vi "Update State String.vi"(8 "error in (no error)":errorcluster, 10 "State Control":string, 11 "Chef State in":refnum<class "Chef State.lvclass">) -> (0 "error out":errorcluster, 3 "Chef State out":refnum<class "Chef State.lvclass">)   [LabVIEW 2021, in "Chef States.lvlib" / "Chef State.lvclass"]
uses:
  Chef State.lvclass
  <vilib>/ActorFramework/Actor/Actor.lvclass
  Root Actor Logic/Root Actor Logic Messages/Update State String Msg/Update State String Msg.lvclass
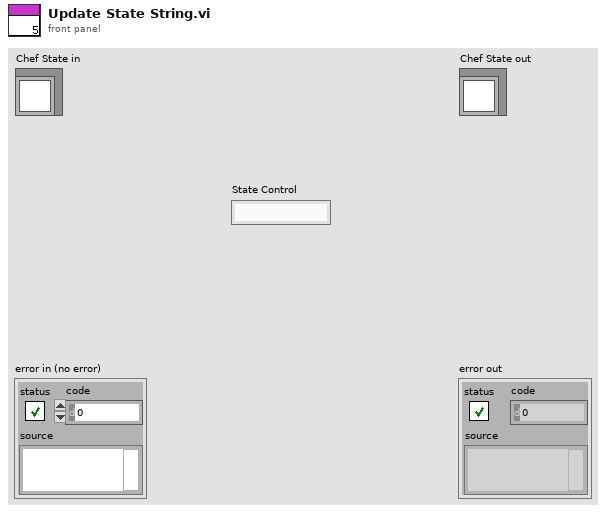
[diagram p1: front panel]
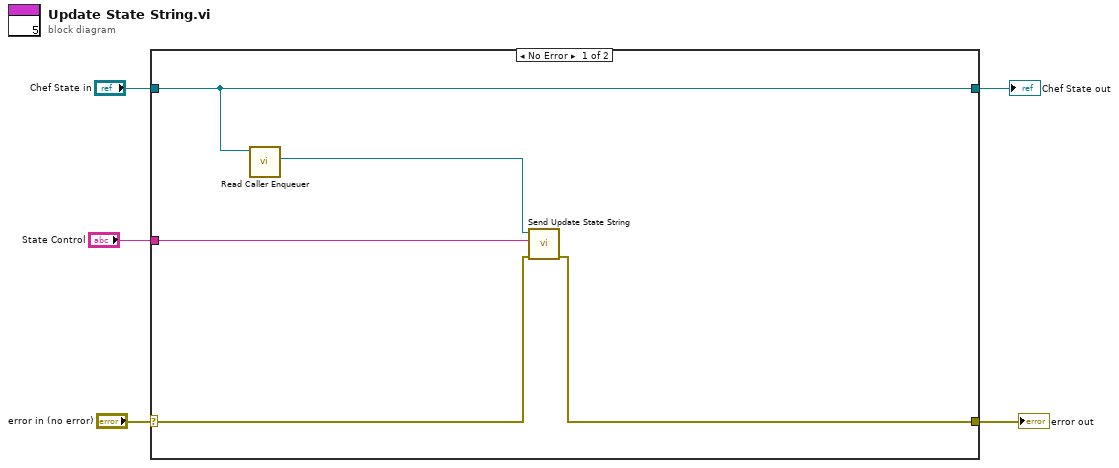
[diagram p0: block diagram]
diagram:
  n1 = case shown="No Error" "error in (no error)" {
    selector: "error in (no error)" -> [w9 w11]
    tunnel: [w8 w11] -> w4
    tunnel: "Chef State in" -> [w10 w12]
    tunnel: [w10 w12] -> w2
    tunnel: "State Control" -> [w7 _]
    frame No Error {
      n2 = call <vilib>:"Read Caller Enqueuer.vi"("Actor"=w10) -> ("Caller Enqueuer"=w6:refnum<class "Message Enqueuer.lvclass">)  [unwired: 10 in]
      n3 = call "Send Update State String.vi"("error in (no error)"=w9, "State"=w7, "Message Enqueuer"=w6) -> ("error out"=w8:errorcluster)  [unwired: 7 in, 1 out]
    }
    frame Error {
    }
  }
  "error out" <- w4
  "Chef State out" <- w2
